vi "GE 5565PIORC.Open.vi"(8 "error in (no error)":errorcluster, 11 "VISA resource name":refnum<visa-resource-name>) -> (0 "error out":errorcluster, 3 "GE 5565PIORC":refnum<class "GE 5565PIORC.lvclass">)   [LabVIEW 2024, in "GE 5565PIORC.lvclass"]
doc: "Opens a new VISA session to the GE Reflective Memory card."
uses:
  GE 5565PIORC.lvclass
  GE 5565PIORC.lvclass/GE 5565PIORC.ctl
  Properties/Registers/GE 5565PIORC.Registers.Local Configuration.Read.vi
  Properties/Registers/GE 5565PIORC.Registers.Local Configuration.Read (U32).vi
  GE 5565PIORC.Registers.Read.vi
  GE 5565PIORC.Registers.Read (U32).vi
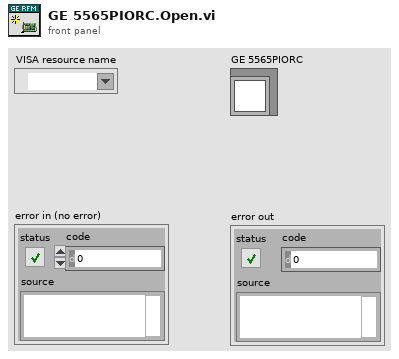
[diagram p1: front panel]
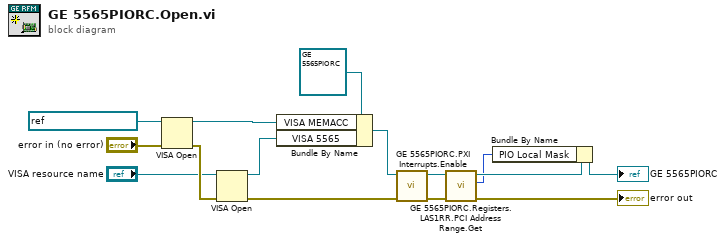
[diagram p0: block diagram]
diagram:
  n1 = VISA Open(error in (no error)="error in (no error)", VISA resource name=refnum<visa-resource-name> "PXI0::MEMACC") -> (VISA resource name=w9:refnum<visa-resource-name>, error out=w7:errorcluster)  [unwired: 3 in]
  n2 = VISA Open(error in (no error)=w7, VISA resource name="VISA resource name") -> (VISA resource name=w6:refnum<visa-resource-name>, error out=w2:errorcluster)  [unwired: 3 in]
  n3 = Bundle By Name(cluster=refnum<class "GE 5565PIORC.lvclass"> refnum ("GE 5565PIORC.lvclass"), "VISA MEMACC"=w9, "VISA 5565"=w6) -> (w1:refnum<class "GE 5565PIORC.lvclass">)
  n4 = call "GE 5565PIORC.PXI Interrupts.Enable.vi"("error in (no error)"=w2, "GE 5565PIORC in"=w1) -> ("error out"=w3:errorcluster, "GE 5565PIORC out"=w4:refnum<class "GE 5565PIORC.lvclass">)  [unwired: 8 in]
  n5 = call "GE 5565PIORC.Registers.LAS1RR.PCI Address Range.Get.vi"("error in (no error)"=w3, "GE 5565PIORC in"=w4) -> ("error out"=→"error out":errorcluster, "PCI Address Range"=w10:u32, "GE 5565PIORC out"=w11:refnum<class "GE 5565PIORC.lvclass">)  [unwired: 7 in]
  n6 = Bundle By Name(cluster=w11, "PIO Local Mask"=w10) -> (→"GE 5565PIORC":refnum<class "GE 5565PIORC.lvclass">)
